vi "FRIC_navX_Internal_I2C_ProcessingLoop.vi"(7 "Device Number":T1, 10 "I2C Bus (in)":T2=enum."I2C MXP", 11 "Update Rate (4Hz-200Hz)":u8=50 min=4 max=200) -> ()   [LabVIEW 2015]
doc: "This navX VI handles the reading/writing for the navX. All of the good stuff is in here.\nTHIS VI SHOULD NOT BE CALLED BY THE USER!"
uses:
  <vilib>/Rock Robotics/SystemInterfaces/i2clib/i2c_bus.ctl
  _TypeDefs/FRIC_navX_DeviceNumbersTypeDef.ctl
  _TypeDefs/FRIC_navX_I2C Process Loop TypeDef.ctl
  _TypeDefs/FRIC_navX_ProcessingLoopStatesTypeDef_I2C.ctl
  _TypeDefs/Z900_navX_DeviceTypeDef.ctl
  _TypeDefs/Z900_navX_ProtocolTypeDef.ctl
  _TypeDefs/Z900_navX_NotifyPacketTypeDef.ctl
  _TypeDefs/Z900_navX_ActionTypeDef.ctl
  _TypeDefs/Z900_navX_SerialStreamTypeDef.ctl
  _TypeDefs/Z900_navX_IntegrationControlRegisters.ctl
  <vilib>/Rock Robotics/WPI/SPI/WPI_SPIDevRef.ctl
  <vilib>/Rock Robotics/SystemInterfaces/spilib/spi_bus.ctl
  _NI WPI Serial USB/WPI_SerialPort_USB.ctl
  <vilib>/Rock Robotics/WPI/SerialPort/WPI_SerialPortRef.ctl
  _TypeDefs/Flags/Z900_navX_Flags_CapabilityTypeDef.ctl
  _TypeDefs/Z900_navX_DeviceRegisters.ctl
  <vilib>/Rock Robotics/SystemInterfaces/Utilities/FPGA_UtilitiesRead LocalTime.vi
  _NI WPI Serial USB/_NI WPI Serial USB.lvlib
panel:
  out "Loop Time (ms)":dbl
  out "Connected":bool
  in  "Halt":bool
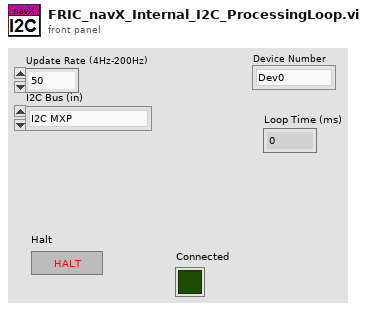
[diagram p1: front panel]
types:
  T1 = typedef "FRIC_navX_DeviceNumbersTypeDef.ctl" = enum16{"Dev0", "Dev1", "Dev2", "Dev3", "Dev4", "Dev5", "Dev6", "Dev7", "Dev8", "Dev9", "Dev10"}
  T2 = typedef "i2c_bus.ctl" = enum16{"I2C On-Board", "I2C MXP", "Invalid"}
  T3 = typedef "FRIC_navX_I2C Process Loop TypeDef.ctl" = cluster{"State Array":T4[], "error":errorcluster, "FPGA Cluster":cluster{"Last Valid FPGA Time":dbl, "Error Count":i32, "Initialized":bool}, "Device Info":T5, "I2CDevRef":cluster{"DevStatus":errorcluster, "Device Address":u8, "Handle":i32, "I2C Bus":T2}, "Registry":u8[], "Command Array":T7[], "Connected?":bool, "navX Device Memory Size":i32, "notification":T8, "Memory Size Set":bool, "SPIDevRef":T11, "navX Serial Open":cluster{"Serial Port":T13, "Stream Type":T10}, "SerialPortRef":T14, "Serial Read Buffer":string, "Serial Write Buffer":string[], "Device Number":T1, "navX SPI Open":cluster{"SPI Bus":T12, "Clock Rate (Hz)":dbl}}
  T4 = typedef "FRIC_navX_ProcessingLoopStatesTypeDef_I2C.ctl" = enum16{"Process", "INI", "Check Packets Valid", "Close", "Flush Serial", "Generate Command", "Last Packet Valid", "Open", "Read", "Reset Serial", "Set Termination Char", "Update AE", "Wait", "Write", "Exit"}
  T5 = typedef "Z900_navX_DeviceTypeDef.ctl" = cluster{"Interface":cluster{"Protocol":T6, "Update Rate (4Hz-200Hz)":u8, "navX Open TypeDef":variant}, "Notify Packet":refnum<notifier>, "Loop VI Refnum":refnum<vi>, "Ready to Close Occurrence Refnum":refnum<k4>, "Name":string}
  T6 = typedef "Z900_navX_ProtocolTypeDef.ctl" = enum16{"SERIAL", "I2C", "SPI"}
  T7 = typedef "Z900_navX_IntegrationControlRegisters.ctl" = u8
  T8 = typedef "Z900_navX_NotifyPacketTypeDef.ctl" = cluster{"navX Action":T9, "Data":variant, "Stream Type":T10}
  T9 = typedef "Z900_navX_ActionTypeDef.ctl" = enum16{"None", "Halt", "Normal Read", "Update Serial Protocol", "Update Rate Htz", "Zero-Yaw", "Zero-Displacement", "Zero-Velocity"}
  T10 = typedef "Z900_navX_SerialStreamTypeDef.ctl" = enum16{"YRPH", "Quaterinons", "Gyro/Raw", "AHRS", "AHRSAndPositioning"}
  T11 = typedef "WPI_SPIDevRef.ctl" = cluster{"DevStatus":errorcluster, "Handle":i32, "SPI Bus":T12}
  T12 = typedef "spi_bus.ctl" = enum16{"SPI On-Board, CS0", "SPI On-Board, CS1", "SPI On-Board, CS2", "SPI On-Board, CS3", "SPI MXP", "Invalid"}
  T13 = typedef "_NI WPI Serial USB.lvlib/WPI_SerialPort_USB.ctl" = enum16{"Onboard RS-232", "MXP TTL", "USB"}
  T14 = typedef "WPI_SerialPortRef.ctl" = cluster{"DevStatus":errorcluster, "Serial Port Name":refnum<visa-resource-name>}
  T15 = typedef "Z900_navX_DeviceRegisters.ctl" = u8
  T16 = typedef "Z900_navX_Flags_CapabilityTypeDef.ctl" = u16
  T17 = cluster{"DevStatus":errorcluster, "Device Address":u8, "Handle":i32, "I2C Bus":T2}
  T18 = cluster{"Last Valid FPGA Time":dbl, "Error Count":i32, "Initialized":bool}
  T19 = typedef "WPI_I2CDevRef.ctl" = cluster{"DevStatus":errorcluster, "Device Address":u8, "Handle":i32, "I2C Bus":T2}
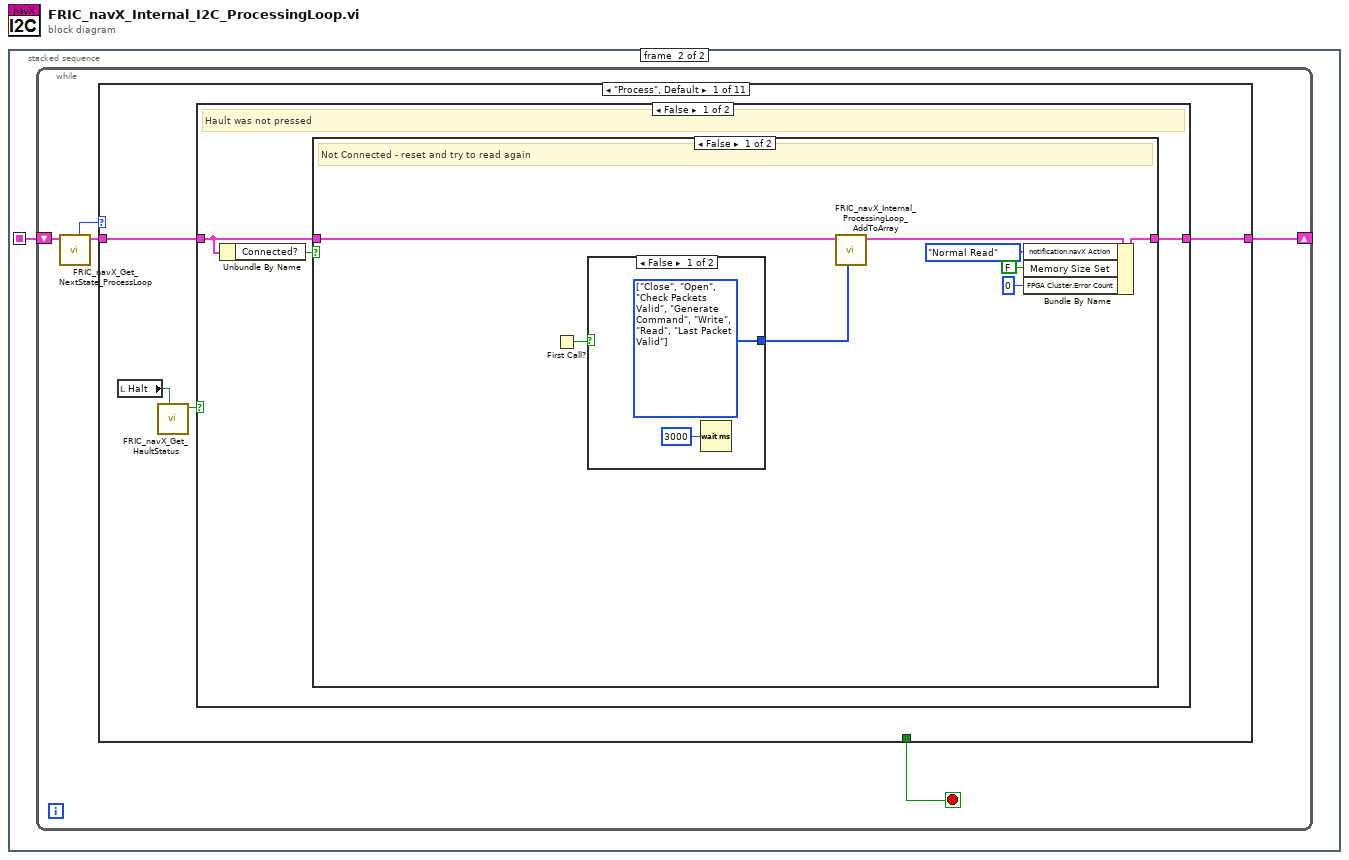
[diagram p0: block diagram]
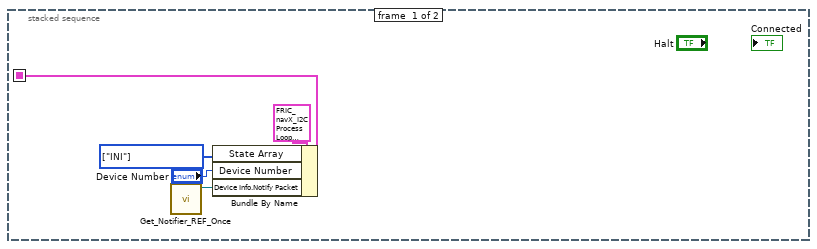
[diagram p2: hidden frame]
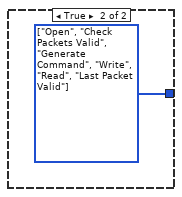
[diagram p3: hidden frame]
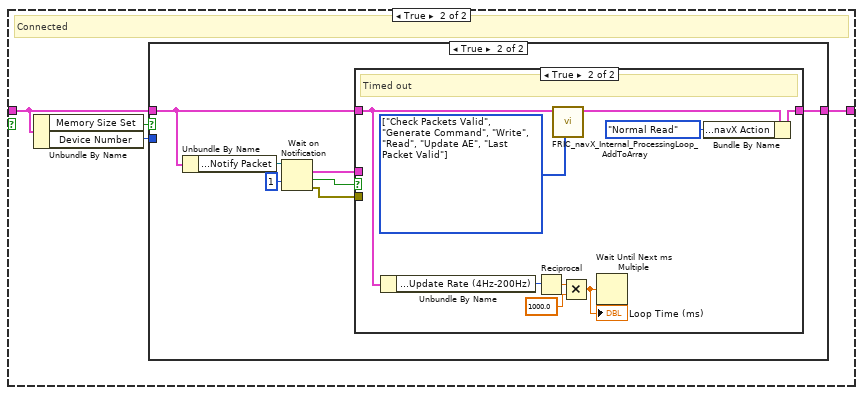
[diagram p4: hidden frame]
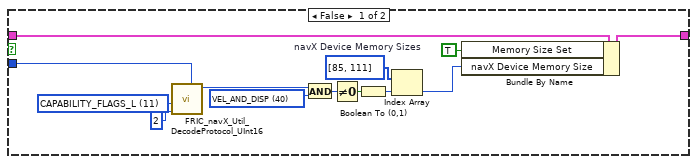
[diagram p5: hidden frame]
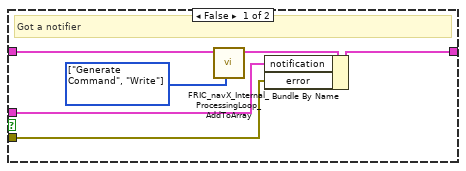
[diagram p6: hidden frame]
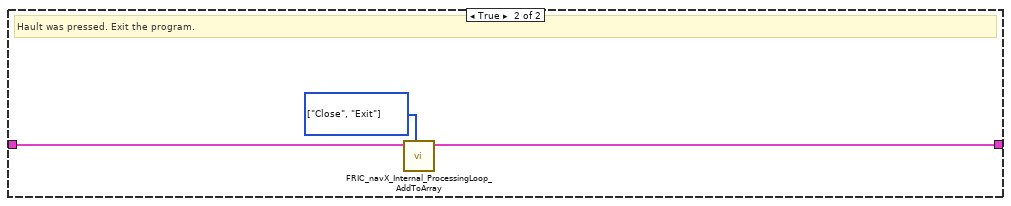
[diagram p7: hidden frame]
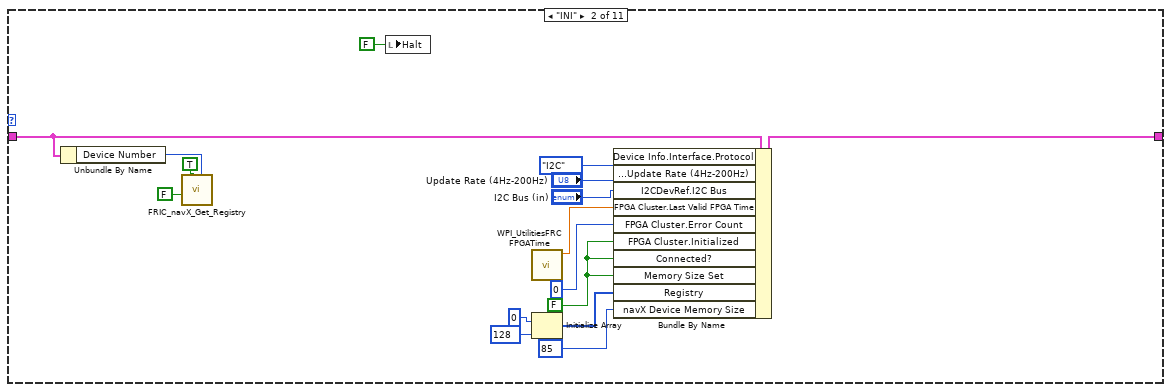
[diagram p8: hidden frame]
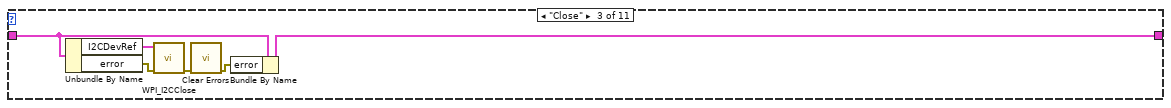
[diagram p9: hidden frame]
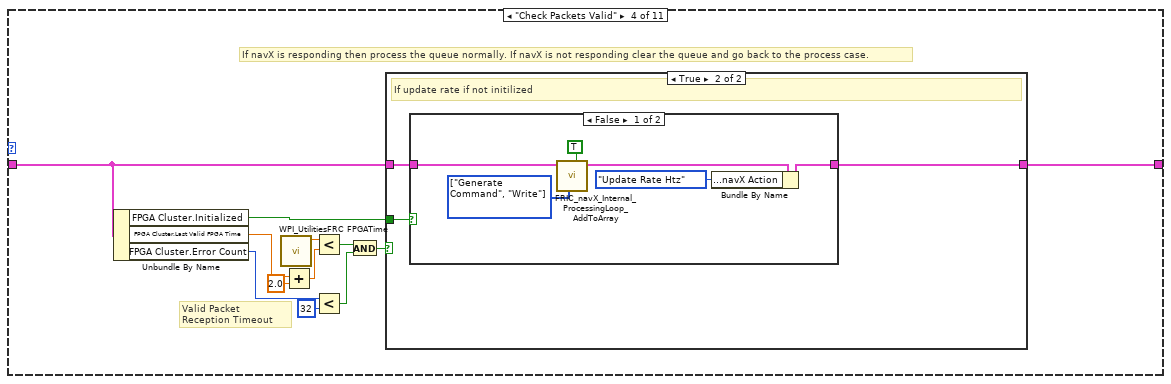
[diagram p10: hidden frame]
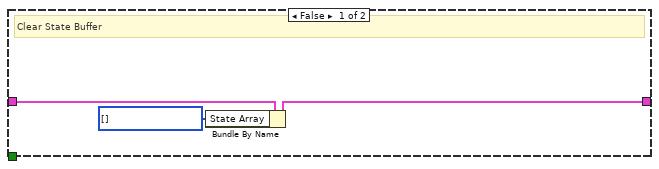
[diagram p11: hidden frame]
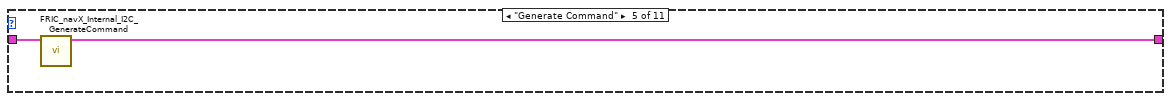
[diagram p13: hidden frame]
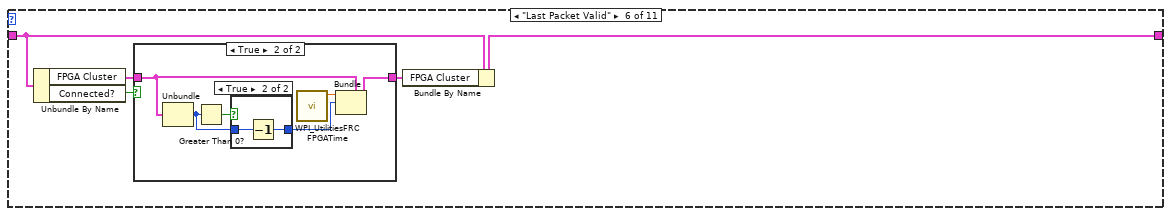
[diagram p14: hidden frame]
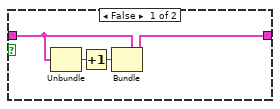
[diagram p15: hidden frame]
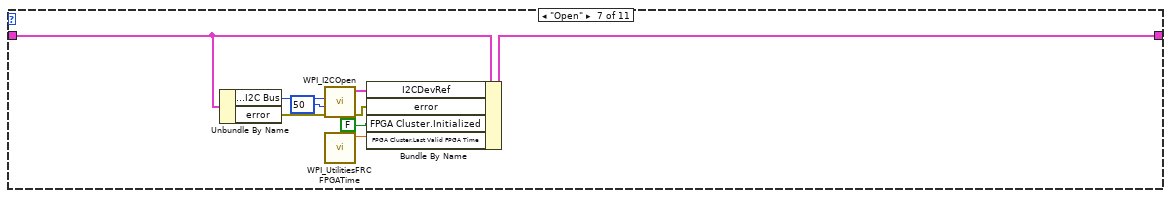
[diagram p17: hidden frame]
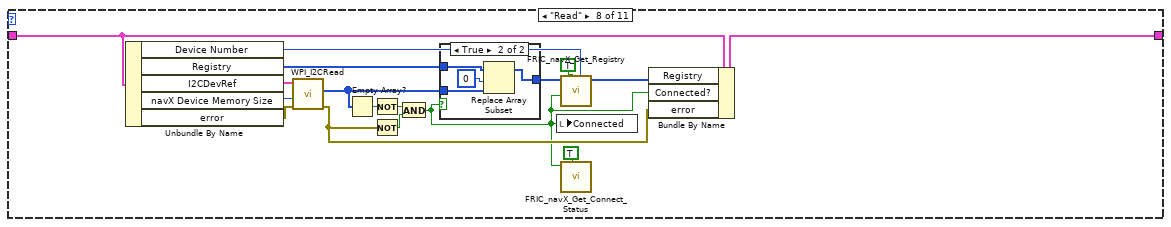
[diagram p18: hidden frame]
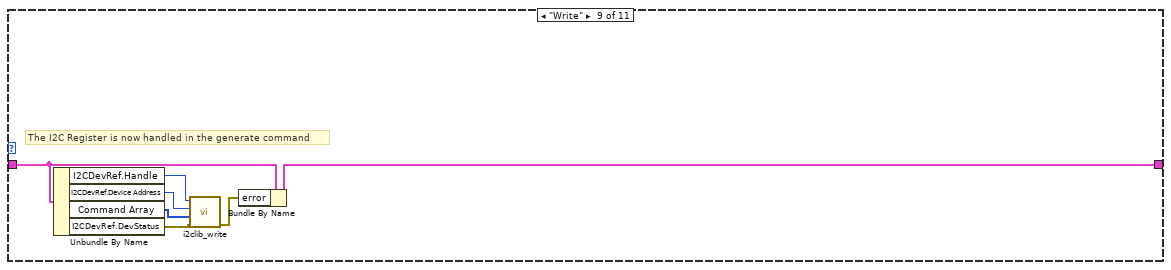
[diagram p20: hidden frame]
diagram:
  n1 = stacked-sequence {
    seq-local: [w5 _] -> [_ w6]
    frame #0 {
      w3 = T4[] [enum."INI"] items=["Process", "INI", "Check Packets Valid", "Close", "Flush Serial", "Generate Command", "Last Packet Valid", "Open", "Read", "Reset Serial", "Set Termination Char", "Update AE", "Wait", "Write", "Exit"] ("State Array")
      n2 = call "Get_Notifier_REF_Once.vi"() -> ("notifier ref out"=w1:refnum<notifier>)  [unwired: 10 in, 1 out]
      n3 = Bundle By Name(cluster=T3 {"State Array"=[enum."INI", enum."Open"], "error"={"status"=FALSE, "code"=0, "source"=""}, "FPGA Cluster"={"Last Valid FPGA Time"=0.0, "Error Count"=0, "Initialized"=FALSE}, "Device Info"={"Interface"={"Protocol"=enum."SERIAL", "Update Rate (4Hz-200Hz)"=4, "navX Open TypeDef"=variant}, "Notify Packet"=refnum, "Loop VI Refnum"=refnum, "Ready to Close Occurrence Refnum"=refnum, "Name"=""}, "I2CDevRef"={"DevStatus"={"status"=FALSE, "code"=0, "source"=""}, "Device Address"=0, "Handle"=0, "I2C Bus"=enum."Invalid"}, "Registry"=[], "Command Array"=[214, 32], "Connected?"=FALSE, "navX Device Memory Size"=85, "notification"={"navX Action"=enum."None", "Data"=variant, "Stream Type"=enum."YRPH"}, "Memory Size Set"=FALSE, "SPIDevRef"={"DevStatus"={"status"=FALSE, "code"=0, "source"=""}, "Handle"=0, "SPI Bus"=enum."SPI On-Board, CS0"}, "navX Serial Open"={"Serial Port"=enum."Onboard RS-232", "Stream Type"=enum."YRPH"}, "SerialPortRef"={"DevStatus"={"status"=FALSE, "code"=0, "source"=""}, "Serial Port Name"=""}, "Serial Read Buffer"="", "Serial Write Buffer"=[], "Device Number"=enum."Dev0", "navX SPI Open"={"SPI Bus"=enum."SPI MXP", "Clock Rate (Hz)"=500000.0}} ("I2C Process Loop TypeDef"), "State Array"=w3, "Device Number"="Device Number", "Device Info.Notify Packet"=w1) -> (w5:T3)
    }
    frame #1 {
      n4 = while {
        shift-right: [w7] -> _
        shift-left: w6 -> [w10]
        stop <- w11 stop-if-true
        n5 = call "FRIC_navX_Get_NextState_ProcessLoop.vi"("I2C Process Loop TypeDef (in)"=w10) -> ("I2C Process Loop TypeDef (out)"=w9:T3, "Current State"=w8:T4)  [unwired: 9 in]
        n6 = case shown="\"Process\", Default" w8 {
          tunnel: [_ _ _ _ _ _ _ _ _ TRUE _] -> w11
          tunnel: w9 -> [w14 w74 w91 w97 w120 w124 w145 w158 w175 w178 w185]
          tunnel: [w15 w80 w90 w98 w119 w123 w144 w157 w176 w178 w185] -> w7
          frame "Process", Default {
            n7 = local read "Halt"() -> (w13:bool)
            n8 = call "FRIC_navX_Get_HaultStatus.vi"("Update"=w13) -> ("Hault"=w12:bool)  [unwired: 10 in]
            n9 = case shown="False" w12 {
              tunnel: [w18 w70] -> w15
              tunnel: w14 -> [w16 w71]
              frame False {
                # "Hault was not pressed"
                n10 = Unbundle By Name(w16) -> ("Connected?"=w17:bool)
                n11 = case shown="False" w17 {
                  tunnel: w16 -> [w26 w32]
                  tunnel: [w23 w33] -> w18
                  frame False {
                    # "Not Connected - reset and try to read again"
                    n12 = First Call?() -> (First Call?: T/F=w19:bool)
                    n13 = case shown="False" w19 {
                      tunnel: [w28 w29] -> w25
                      frame False {
                        w28 = T4[] [enum."Close", enum."Open", enum."Check Packets Valid", enum."Generate Command", enum."Write", enum."Read", enum."Last Packet Valid"] items=["Process", "INI", "Check Packets Valid", "Close", "Flush Serial", "Generate Command", "Last Packet Valid", "Open", "Read", "Reset Serial", "Set Termination Char", "Update AE", "Wait", "Write", "Exit"]
                        n14 = Wait (ms)(milliseconds to wait=u32 3000) -> ()  [unwired: 1 out]
                      }
                      frame True {
                        w29 = T4[] [enum."Open", enum."Check Packets Valid", enum."Generate Command", enum."Write", enum."Read", enum."Last Packet Valid"] items=["Process", "INI", "Check Packets Valid", "Close", "Flush Serial", "Generate Command", "Last Packet Valid", "Open", "Read", "Reset Serial", "Set Termination Char", "Update AE", "Wait", "Write", "Exit"]
                      }
                    }
                    n15 = call "FRIC_navX_Internal_ProcessingLoop_AddToArray.vi"("States Array"=w25, "I2C Process Loop TypeDef (in)"=w26) -> ("I2C Process Loop TypeDef (out)"=w24:T3)  [unwired: 9 in]
                    n16 = Bundle By Name(cluster=w24, "notification.navX Action"=Z900_navX_ActionTypeDef."Normal Read", "Memory Size Set"=FALSE, "FPGA Cluster.Error Count"=0) -> (w23:T3)
                  }
                  frame True {
                    # "Connected"
                    n17 = Unbundle By Name(w32) -> ("Memory Size Set"=w31:bool, "Device Number"=w30:T1)
                    n18 = case shown="True" w31 {
                      tunnel: [w45 w51] -> w33
                      tunnel: w32 -> [w46 w48]
                      tunnel: w30 -> [w34 _]
                      frame False {
                        w44 = T15 11 items=["WHOAMI"=0, "HW_REV"=1, "FW_VER_MAJOR"=2, "FW_VER_MINOR"=3, "UPDATE_RATE_HZ"=4, "ACCEL_FSR_G"=5, "GYRO_FSR_DPS"=6, "OP_STATUS"=8, "CAL_STATUS"=9, "SELFTEST_STATUS"=10, "CAPABILITY_FLAGS_L"=11, "CAPABILITY_FLAGS_H"=12, "SENSOR_STATUS"=16, "TIMESTAMP"=18, "YAW"=22, "ROLL"=24, "PITCH"=26, "HEADING"=28, "FUSED_HEADING"=30, "ALTITUDE_I"=32, "ALTITUDE_D"=34, "LINERA_ACC_X"=36, "LINERA_ACC_Y"=38, "LINERA_ACC_Z"=40, "QUAT_W"=42, "QUAT_X"=44, "QUAT_Y"=46, "QUAT_Z"=48, "MPU_TEMP_C"=50, "GYRO_X"=52, "GYRO_Y"=54, "GYRO_Z"=56, "ACC_X"=58, "ACC_Y"=60, "ACC_Z"=62, "MAG_X"=64, "MAG_Y"=66, "MAG_Z"=68, "PRESSURE_I"=70, "PRESSURE_D"=72, "PRESSURE_TEMP"=74, "YAW_OFFSET"=76, "QUAT_OFFSET_W"=78, "QUAT_OFFSET_X"=80, "QUAT_OFFSET_Y"=82, "QUAT_OFFSET_Z"=84, "INTEGRATION_CONTROL"=86, "VELOCITY_X"=88, "VELOCITY_Y"=92, "VELOCITY_Z"=96, "DISPLACMENT_X"=100, "DISPLACMENT_Y"=104, "DISPLACEMENT_Z"=108] ("Device Register")
                        w39 = T16 40 items=["OMNIMOUNT"=4, "OMNIMOUNT_CONFIG_MASK"=38, "VEL_AND_DISP"=40, "YAW_RESET"=80] ("Capability Flag")
                        w40 = i32[] [85, 111]  # navX Device Memory Sizes
                        n19 = call "FRIC_navX_Util_DecodeProtocol_UInt16.vi"("Device Number"=w34, "length"=2, "Device Register"=w44) -> ("Value"=w37:u16)  [unwired: 8 in]
                        n20 = And(x=w37, y=w39) -> (x .and. y?=w38:T16)
                        n21 = Not Equal To 0?(x=w38) -> (x != 0?=w41:bool)
                        n22 = Boolean To (0,1)(Boolean=w41) -> (0, 1=w42:i16)
                        n23 = Index Array(array=w40, index=w42) -> (element=w36:i32)
                        n24 = Bundle By Name(cluster=w46, "Memory Size Set"=TRUE, "navX Device Memory Size"=w36) -> (w45:T3)
                      }
                      frame True {
                        n25 = Unbundle By Name(w48) -> ("Device Info.Notify Packet"=w53:refnum<notifier>)
                        n26 = Wait on Notification(notifier=w53, timeout in ms (-1)=1) -> (notification=w50:T8, timed out?=w47:bool, error out=w49:errorcluster)  [unwired: 2 in, 1 out]
                        n27 = case shown="True" w47 {
                          tunnel: w48 -> [w59 w60]
                          tunnel: [w58 w66] -> w51
                          tunnel: w50 -> [w57 _]
                          tunnel: w49 -> [w54 _]
                          frame False {
                            w55 = T4[] [enum."Generate Command", enum."Write"] items=["Process", "INI", "Check Packets Valid", "Close", "Flush Serial", "Generate Command", "Last Packet Valid", "Open", "Read", "Reset Serial", "Set Termination Char", "Update AE", "Wait", "Write", "Exit"] ("States Array")
                            # "Got a notifier"
                            n28 = call "FRIC_navX_Internal_ProcessingLoop_AddToArray.vi"("States Array"=w55, "I2C Process Loop TypeDef (in)"=w59) -> ("I2C Process Loop TypeDef (out)"=w56:T3)  [unwired: 9 in]
                            n29 = Bundle By Name(cluster=w56, "notification"=w57, "error"=w54) -> (w58:T3)
                          }
                          frame True {
                            w68 = T4[] [enum."Check Packets Valid", enum."Generate Command", enum."Write", enum."Read", enum."Update AE", enum."Last Packet Valid"] items=["Process", "INI", "Check Packets Valid", "Close", "Flush Serial", "Generate Command", "Last Packet Valid", "Open", "Read", "Reset Serial", "Set Termination Char", "Update AE", "Wait", "Write", "Exit"]
                            # "Timed out"
                            n30 = Unbundle By Name(w60) -> ("Device Info.Interface.Update Rate (4Hz-200Hz)"=w61:u8)
                            n31 = Reciprocal(x=w61) -> (1/x=w62:dbl)
                            n32 = call "FRIC_navX_Internal_ProcessingLoop_AddToArray.vi"("States Array"=w68, "I2C Process Loop TypeDef (in)"=w60) -> ("I2C Process Loop TypeDef (out)"=w67:T3)  [unwired: 9 in]
                            n33 = Multiply(x=w62, y=1000.0) -> (x*y=w64:dbl)
                            "Loop Time (ms)" <- w64
                            n34 = Wait Until Next ms Multiple(millisecond multiple=w64) -> ()  [unwired: 1 out]
                            n35 = Bundle By Name(cluster=w67, "notification.navX Action"=Z900_navX_ActionTypeDef."Normal Read") -> (w66:T3)
                          }
                        }
                      }
                    }
                  }
                }
              }
              frame True {
                w69 = T4[] [enum."Close", enum."Exit"] items=["Process", "INI", "Check Packets Valid", "Close", "Flush Serial", "Generate Command", "Last Packet Valid", "Open", "Read", "Reset Serial", "Set Termination Char", "Update AE", "Wait", "Write", "Exit"] ("States Array")
                # "Hault was pressed. Exit the program."
                n36 = call "FRIC_navX_Internal_ProcessingLoop_AddToArray.vi"("States Array"=w69, "I2C Process Loop TypeDef (in)"=w71) -> ("I2C Process Loop TypeDef (out)"=w70:T3)  [unwired: 9 in]
              }
            }
          }
          frame "INI" {
            w78 = FALSE ("Initialized")
            n37 = Unbundle By Name(w74) -> ("Device Number"=w73:T1)
            n38 = call "FRIC_navX_Get_Registry.vi"("Device Number"=w73, "Update"=TRUE, "Connected?"=FALSE) -> ()  [unwired: 7 in, 2 out]
            n39 = local write "Halt"(FALSE ("Halt")) -> ()
            n40 = call <vilib>:"WPI_UtilitiesFRC FPGATime.vi"() -> ("FPGA Time"=w82:dbl)  [unwired: 10 in, 1 out]
            n41 = Initialize Array(u8 0 ("Received Data"), 128 ("hex")) -> (w77:u8[])
            n42 = Bundle By Name(cluster=w74, "Device Info.Interface.Protocol"=Z900_navX_ProtocolTypeDef."I2C" ("Protocol"), "Device Info.Interface.Update Rate (4Hz-200Hz)"="Update Rate (4Hz-200Hz)", "I2CDevRef.I2C Bus"="I2C Bus (in)", "FPGA Cluster.Last Valid FPGA Time"=w82, "FPGA Cluster.Error Count"=0 ("Error Count"), "FPGA Cluster.Initialized"=w78, "Connected?"=w78, "Memory Size Set"=w78, "Registry"=w77, "navX Device Memory Size"=85 ("hex")) -> (w80:T3)
          }
          frame "Close" {
            n43 = Unbundle By Name(w91) -> ("I2CDevRef"=w93:T17, "error"=w92:errorcluster)
            n44 = call <vilib>:"WPI_I2CClose.vi"("error in (no error)"=w92, "I2CDevRef"=w93) -> ("error out"=w89:errorcluster)  [unwired: 9 in]
            n45 = call <vilib>:"Clear Errors.vi"("error in (no error)"=w89) -> ("error out"=w88:errorcluster)  [unwired: 5 in, 1 out]
            n46 = Bundle By Name(cluster=w91, "error"=w88) -> (w90:T3)
          }
          frame "Check Packets Valid" {
            # "If navX is responding then process the queue normally. If navX is not responding clear the queue and go back to the process case."
            # "Valid Packet Reception Timeout"
            n47 = Unbundle By Name(w97) -> ("FPGA Cluster.Initialized"=w95:bool, "FPGA Cluster.Last Valid FPGA Time"=w96:dbl, "FPGA Cluster.Error Count"=w94:i32)
            n48 = call <vilib>:"WPI_UtilitiesFRC FPGATime.vi"() -> ("FPGA Time"=w103:dbl)  [unwired: 10 in, 1 out]
            n49 = Add(x=w96, y=2.0) -> (x+y=w104:dbl)
            n50 = Less?(x=w103, y=w104) -> (x < y?=w101:bool)
            n51 = Less?(x=w94, y=32) -> (x < y?=w100:bool)
            n52 = And(x=w101, y=w100) -> (x .and. y?=w99:bool)
            n53 = case shown="True" w99 {
              tunnel: w97 -> [w108 w111]
              tunnel: [w107 w110] -> w98
              tunnel: w95 -> [_ w109]
              frame False {
                w106 = T4[] [] items=["Process", "INI", "Check Packets Valid", "Close", "Flush Serial", "Generate Command", "Last Packet Valid", "Open", "Read", "Reset Serial", "Set Termination Char", "Update AE", "Wait", "Write", "Exit"] ("f")
                # "Clear State Buffer"
                n54 = Bundle By Name(cluster=w108, "State Array"=w106) -> (w107:T3)
              }
              frame True {
                # "If update rate if not initilized"
                n55 = case shown="False" w109 {
                  tunnel: w111 -> [w116 w118]
                  tunnel: [w114 w118] -> w110
                  frame False {
                    w112 = T4[] [enum."Generate Command", enum."Write"] items=["Process", "INI", "Check Packets Valid", "Close", "Flush Serial", "Generate Command", "Last Packet Valid", "Open", "Read", "Reset Serial", "Set Termination Char", "Update AE", "Wait", "Write", "Exit"] ("f")
                    n56 = call "FRIC_navX_Internal_ProcessingLoop_AddToArray.vi"("Add to beginning"=TRUE, "States Array"=w112, "I2C Process Loop TypeDef (in)"=w116) -> ("I2C Process Loop TypeDef (out)"=w115:T3)  [unwired: 8 in]
                    n57 = Bundle By Name(cluster=w115, "notification.navX Action"=Z900_navX_ActionTypeDef."Update Rate Htz") -> (w114:T3)
                  }
                  frame True {
                  }
                }
              }
            }
          }
          frame "Generate Command" {
            n58 = call "FRIC_navX_Internal_I2C_GenerateCommand.vi"("I2C Process Loop TypeDef (in)"=w120) -> ("I2C Process Loop TypeDef (out)"=w119:T3)  [unwired: 10 in]
          }
          frame "Last Packet Valid" {
            n59 = Unbundle By Name(w124) -> ("FPGA Cluster"=w125:T18, "Connected?"=w121:bool)
            n60 = case shown="True" w121 {
              tunnel: [w128 w135] -> w122
              tunnel: w125 -> [w127 w131]
              frame False {
                n61 = Unbundle(w127) -> ("Error Count"=w126:i32)  [unwired: 2 out]
                n62 = Increment(x=w126) -> (x+1=w129:i32)
                n63 = Bundle(cluster=w127, "Error Count"=w129) -> (w128:T18)  [unwired: 2 in]
              }
              frame True {
                n64 = Unbundle(w131) -> ("Error Count"=w130:i32)  [unwired: 2 out]
                n65 = Greater Than 0?(x=w130) -> (x > 0?=w133:bool)
                n66 = case shown="True" w133 {
                  tunnel: [w136 w138] -> w132
                  tunnel: w130 -> [w136 w137]
                  frame False {
                  }
                  frame True {
                    n67 = Decrement(x=w137) -> (x-1=w138:i32)
                  }
                }
                n68 = call <vilib>:"WPI_UtilitiesFRC FPGATime.vi"() -> ("FPGA Time"=w134:dbl)  [unwired: 10 in, 1 out]
                n69 = Bundle(cluster=w131, "Last Valid FPGA Time"=w134, "Error Count"=w132) -> (w135:T18)  [unwired: 1 in]
              }
            }
            n70 = Bundle By Name(cluster=w124, "FPGA Cluster"=w122) -> (w123:T3)
          }
          frame "Open" {
            n71 = Unbundle By Name(w145) -> ("I2CDevRef.I2C Bus"=w139:T2, "error"=w140:errorcluster)
            n72 = call <vilib>:"WPI_I2COpen.vi"("error in"=w140, "Device Address"=u8 50, "I2C Bus"=w139) -> ("error out"=w143:errorcluster, "I2CDevRef"=w146:T19)  [unwired: 7 in]
            n73 = call <vilib>:"WPI_UtilitiesFRC FPGATime.vi"() -> ("FPGA Time"=w141:dbl)  [unwired: 10 in, 1 out]
            n74 = Bundle By Name(cluster=w145, "I2CDevRef"=w146, "error"=w143, "FPGA Cluster.Initialized"=FALSE ("Initialized"), "FPGA Cluster.Last Valid FPGA Time"=w141) -> (w144:T3)
          }
          frame "Read" {
            n75 = Unbundle By Name(w158) -> ("Device Number"=w153:T1, "Registry"=w154:u8[], "I2CDevRef"=w161:T17, "navX Device Memory Size"=w159:i32, "error"=w160:errorcluster)
            n76 = call <vilib>:"WPI_I2CRead.vi"("error in (no error)"=w160, "I2CBytesToRead"=w159, "I2CDevRef"=w161) -> ("error out"=w155:errorcluster, "Data Out"=w152:u8[])  [unwired: 6 in, 1 out]
            n77 = Empty Array?(array=w152) -> (empty?=w151:bool)
            n78 = Not(x=w151) -> (.not. x?=w150:bool)
            n79 = Not(x=w155) -> (.not. x?=w162:bool)
            n80 = And(x=w150, y=w162) -> (x .and. y?=w149:bool)
            n81 = case shown="True" w149 {
              tunnel: w154 -> [w165 w169]
              tunnel: [w165 w168] -> w164
              tunnel: w152 -> [_ w167]
              frame False {
              }
              frame True {
                n82 = Replace Array Subset(array=w169, new element=w167, index=u8 0 ("hex")) -> (w168:u8[])
              }
            }
            n83 = local write "Connected"(w149) -> ()
            n84 = call "FRIC_navX_Get_Registry.vi"("Device Number"=w153, "Update"=TRUE, "Connected?"=w149, "Registry (in)"=w164) -> ("Registry (out)"=w156:u8[])  [unwired: 6 in, 1 out]
            n85 = call "FRIC_navX_Get_Connect_Status.vi"("Update"=TRUE, "Connected"=w149) -> ()  [unwired: 9 in, 1 out]
            n86 = Bundle By Name(cluster=w158, "Registry"=w156, "Connected?"=w149, "error"=w155) -> (w157:T3)
          }
          frame "Write" {
            # "The I2C Register is now handled in the generate command"
            n87 = Unbundle By Name(w175) -> ("I2CDevRef.Handle"=w174:i32, "I2CDevRef.Device Address"=w173:u8, "Command Array"=w171:T7[], "I2CDevRef.DevStatus"=w172:errorcluster)
            n88 = call <vilib>:"i2clib_write.vi"("error in (no error)"=w172, "send_data"=w171, "dev_addr"=w173, "I2C Reference"=w174) -> ("error out"=w170:errorcluster)  [unwired: 6 in, 1 out]
            n89 = Bundle By Name(cluster=w175, "error"=w170) -> (w176:T3)
          }
          frame "Exit" {
            n90 = Unbundle By Name(w178) -> ("Device Info"=w177:T5)
            n91 = in-place {
              in-place-border: w177 -> [w181]
              in-place-border: [TRUE] -> w180
              # "Set Occurence of Close"
              n92 = Unbundle By Name(w181) -> ("Ready to Close Occurrence Refnum"=w183:refnum<k4>)
              n93 = local write "Halt"(FALSE ("Halt")) -> ()
              n94 = Set Occurrence(w183) -> ()
            }
            n95 = Stop(stop? (T)=w180) -> ()
          }
          frame "Update AE" {
            n96 = Unbundle By Name(w185) -> ("Device Number"=w186:T1)
            n97 = call "FRIC_navX_Internal_ProcessingLoop_UpdateAE.vi"("Device Number"=w186) -> ()  [unwired: 5 in, 10 out]
          }
        }
      }
    }
  }
